vi "GA Crd Status.vi"(7 "FifoIndex":i16, 8 "error in (no error)":errorcluster caption="错误输入（无错误）", 9 "pSegment":i32, 10 "pRun":i16, 11 "nCrdNum":i16) -> (0 "error out":errorcluster caption="错误输出", 1 "pSegment out":i32, 2 "pRun out":i16, 3 "function return":i32)   [LabVIEW 2015, in "GAS.lvlib"]
doc: "extern \"C\" __declspec(dllimport) int GA_CrdStatus(short nCrdNum,short *pRun,long *pSegment,short FifoIndex=0);"
uses:
  <userlib>/BP_GAS/GAS.lvlib
  <userlib>/BP_GAS/GAS.dll
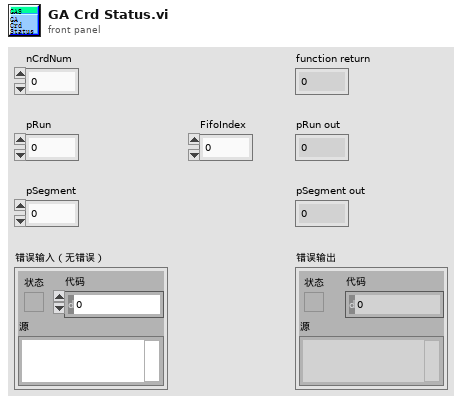
[diagram p1: front panel]
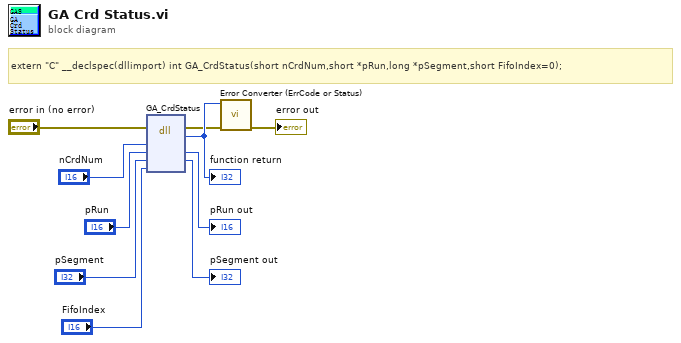
[diagram p0: block diagram]
diagram:
  # "extern \"C\" __declspec(dllimport) int GA_CrdStatus(short nCrdNum,short *pRun,long *pSegment,short FifoIndex=0);"
  n1 = dll-call lib="E:/Program Files (x86)/National Instruments/LabVIEW 2015/user.lib/BP_GAS/GAS.*" fn="GA_CrdStatus"(error in="error in (no error)", "nCrdNum"="nCrdNum", "pRun"="pRun", "pSegment"="pSegment", "FifoIndex"="FifoIndex") -> (error out=w2:errorcluster, w10:i32, "pRun"=→"pRun out":i16, "pSegment"=→"pSegment out":i32)  [unwired: 4 in, 1 out]
  "function return" <- w10
  n2 = call "Error Converter (ErrCode or Status).vi"("error in (no error)"=w2, "error code"=w10) -> ("error out"=→"error out":errorcluster)  [unwired: 9 in]
